vi "mapV4.vi"() -> ()   [LabVIEW 2024]
uses:
  D:/Autonomous Systems/Oulu/Measurment Systems/EnvironmentalMonitoringSystem/GMapControl/GMapControl/bin/Debug/GMapControl.dll
  GMapControl/GMapControl/bin/Debug/GMapControl.dll
panel:
  out "GetLastAction":i32
  out "id_list":u16[](array[numeric])
  out "GetLongitude":dbl
  out "GetLatitude":dbl
  out "Button":u16
  out "mouse event":bool
  in  "MapControl":refnum<k24>(container)
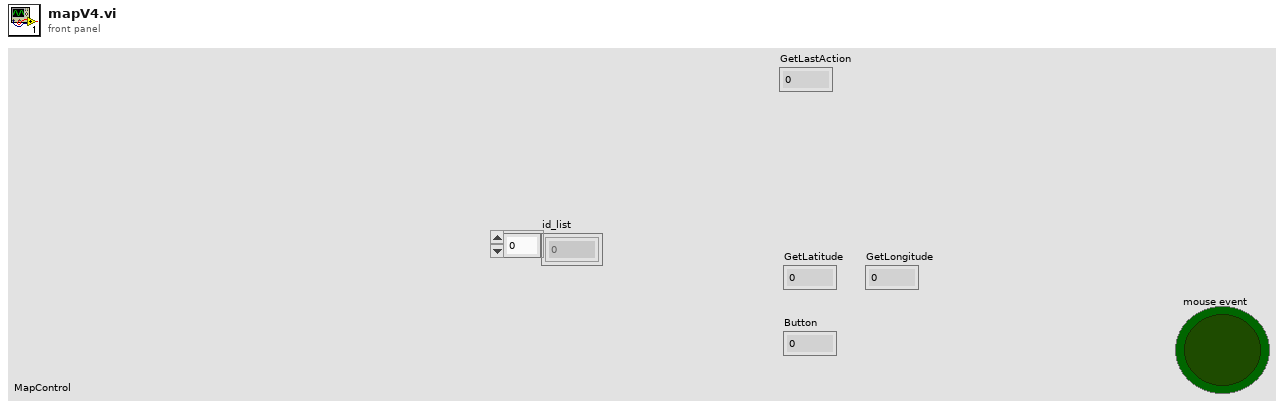
[diagram p1: front panel]
types:
  T1 = cluster{"meta":cluster{"name":string, "website":string, "page":dbl, "limit":dbl}, "results":cluster{"id":i32, "name":string, "distance":dbl, "coordinates":cluster{"latitude":dbl, "longitude":dbl}}[]}
  T2 = cluster{"id":i32, "name":string, "distance":dbl, "coordinates":cluster{"latitude":dbl, "longitude":dbl}}[]
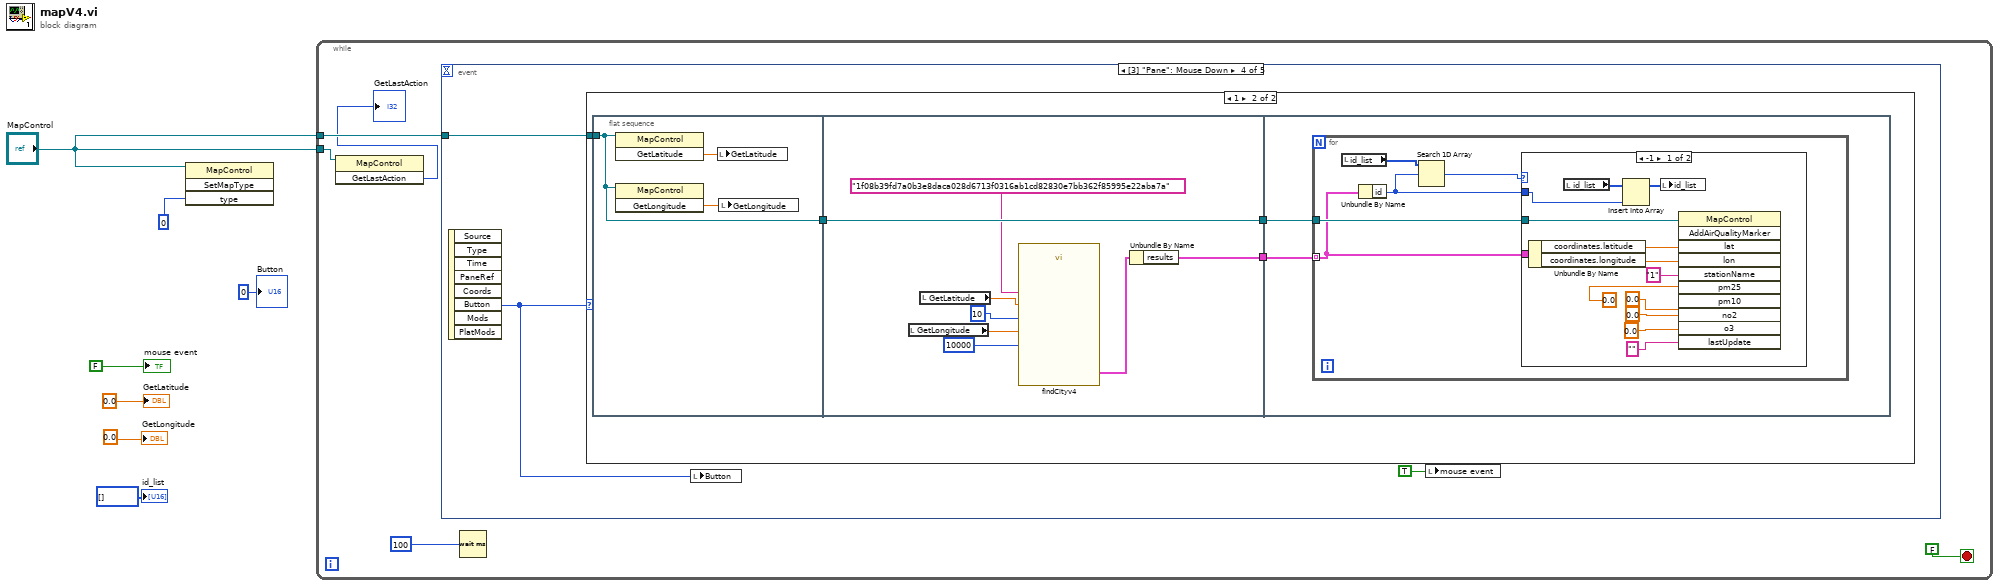
[diagram p0: block diagram]
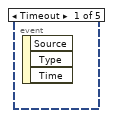
[diagram p2: hidden frame]
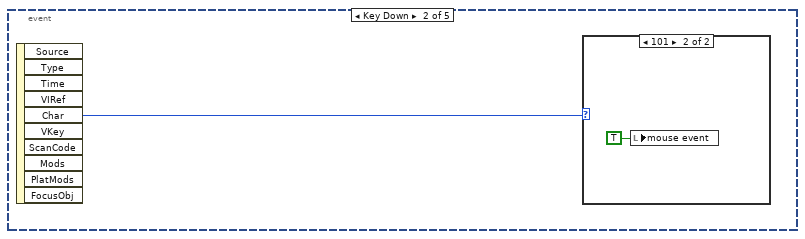
[diagram p3: hidden frame]
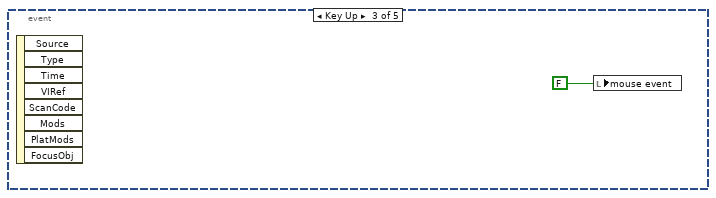
[diagram p5: hidden frame]
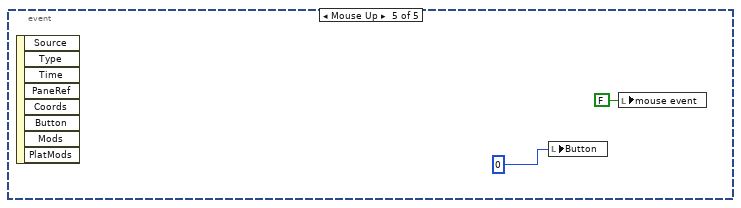
[diagram p8: hidden frame]
diagram:
  n1 = invoke class="MapControl" method="SetMapType"(reference="MapControl", "type"=0) -> ()  [unwired: 2 in, 4 out]
  n2 = while {
    tunnel: "MapControl" -> [w10]
    tunnel: "MapControl" -> [w9]
    stop <- FALSE stop-if-true
    n3 = invoke class="MapControl" method="GetLastAction"(reference=w9) -> ("GetLastAction"=→"GetLastAction":i32)  [unwired: 2 in, 2 out]
    n4 = event shown="[3] \"Pane\": Mouse Down" {
      selector: _ -> [_ _ _ _ _]
      dyn-events: _ -> [_ _ _ _ _]
      timeout: _ -> [_ _ _ _ _]
      tunnel: w10 -> [_ _ _ w17 _]
      event Timeout {
        n5 = event-data() -> ()  [unwired: 1 in, 3 out]
      }
      event Key Down {
        n6 = event-data() -> ("Char"=w13:i16)  [unwired: 1 in, 9 out]
        n7 = case shown="101" w13 {
          frame Default {
          }
          frame 101 {
            n8 = local write "mouse event"(TRUE ("mouse event")) -> ()
          }
        }
      }
      event Key Up {
        n9 = event-data() -> ()  [unwired: 1 in, 8 out]
        n10 = local write "mouse event"(FALSE ("mouse event")) -> ()
      }
      event Mouse Down {
        n11 = event-data() -> ("Button"=w16:u16)  [unwired: 1 in, 7 out]
        n12 = case shown="1" w16 {
          tunnel: w17 -> [_ w22]
          frame Default {
          }
          frame 1 {
            n13 = flat-sequence {
              tunnel: w22 -> [w23]
              tunnel: [w23] -> w21
              tunnel: w21 -> [w33]
              tunnel: [w33] -> w20
              tunnel: [w32] -> w19
              tunnel: w20 -> [w35]
              tunnel: w19 -> [w34]
              frame #0 {
                n14 = invoke class="MapControl" method="GetLatitude"(reference=w23) -> ("GetLatitude"=w25:dbl)  [unwired: 2 in, 2 out]
                n15 = invoke class="MapControl" method="GetLongitude"(reference=w23) -> ("GetLongitude"=w24:dbl)  [unwired: 2 in, 2 out]
                n16 = local write "GetLatitude"(w25) -> ()
                n17 = local write "GetLongitude"(w24) -> ()
              }
              frame #1 {
                n18 = local read "GetLongitude"() -> (w29:dbl)
                n19 = local read "GetLatitude"() -> (w27:dbl)
                n20 = call "findCityv4.vi"("limit"=u16 10, "API-key"="1f08b39fd7a0b3e8daca028d6713f0316ab1cd82830e7bb362f85995e22aba7a", "longitude"=w29, "latitude"=w27, "range"=u16 10000) -> ("value"=w31:T1)  [unwired: 1 out]
                n21 = Unbundle By Name(w31) -> ("results"=w32:T2)
              }
              frame #2 {
                n22 = for {
                  tunnel: w35 -> [w40]
                  tunnel: w34 -> [w39] mode=indexing
                  n23 = local read "id_list"() -> (w38:u16[])
                  n24 = Unbundle By Name(w39) -> ("id"=w36:i32)
                  n25 = Search 1D Array(1D array=w38, element=w36) -> (index of element=w37:i32)  [unwired: 1 in]
                  n26 = case shown="-1" w37 {
                    tunnel: w40 -> [w53 _]
                    tunnel: w39 -> [w44 _]
                    tunnel: w36 -> [w41 _]
                    frame -1 {
                      n27 = Unbundle By Name(w44) -> ("coordinates.latitude"=w46:dbl, "coordinates.longitude"=w45:dbl)
                      n28 = local read "id_list"() -> (w42:u16[])
                      n29 = Insert Into Array(array=w42, new element=w41) -> (w43:u16[])  [unwired: 1 in]
                      n30 = local write "id_list"(w43) -> ()
                      n31 = invoke class="MapControl" method="AddAirQualityMarker"(reference=w53, "lat"=w46, "lon"=w45, "stationName"="1", "pm25"=0.0, "pm10"=0.0, "no2"=0.0, "o3"=0.0, "lastUpdate"="") -> ()  [unwired: 2 in, 11 out]
                    }
                    frame Default {
                    }
                  }
                }
              }
            }
          }
        }
        n32 = local write "Button"(w16) -> ()
        n33 = local write "mouse event"(TRUE ("mouse event")) -> ()
      }
      event Mouse Up {
        n34 = event-data() -> ()  [unwired: 1 in, 8 out]
        n35 = local write "Button"(u16 0 ("Button")) -> ()
        n36 = local write "mouse event"(FALSE ("mouse event")) -> ()
      }
    }
    n37 = Wait (ms)(milliseconds to wait=u32 100) -> ()  [unwired: 1 out]
  }
  "mouse event" <- FALSE ("mouse event")
  "Button" <- u16 0 ("Button")
  "GetLatitude" <- 0.0 ("GetLatitude")
  "GetLongitude" <- 0.0 ("GetLongitude")
  "id_list" <- u16[] [] ("id_list")
